vi "View.vi"(0 "object in":refnum<class "Excel.lvclass">, 2 "Requirements":T2, 5 "Error In":errorcluster) -> (14 "object out":refnum<class "Excel.lvclass">, 16 "Message":T1, 19 "Error Out":errorcluster)   [LabVIEW 2024, in "Excel.lvclass"]
doc: "Opens an Excel file and runs Viewer classes Execute method"
uses:
  Excel.lvclass
  Support/Type Def/Requirements.ctl
  Support/Type Def/File Type.ctl
  Support/Type Def/Message.ctl
  IDataMethod_interface/IDataMethod.lvclass
panel:
  # "Connector Pane"
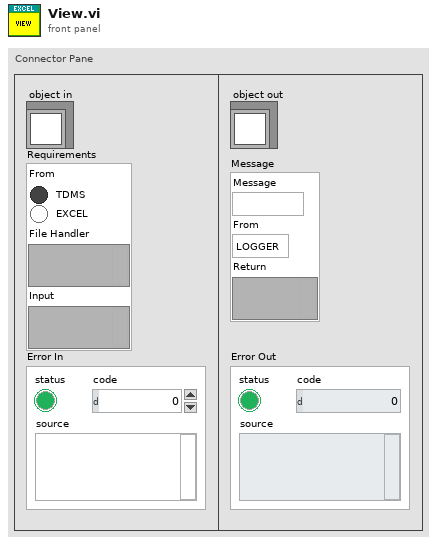
[diagram p1: front panel]
types:
  T1 = typedef "Message.ctl" = cluster{"Message":string, "From":enum16{"LOGGER", "VIEWER"}, "Return":variant}
  T2 = typedef "Requirements.ctl" = cluster{"From":T3, "File Handler":variant, "Input":variant}
  T3 = typedef "File Type.ctl" = enum32{"TDMS", "EXCEL"}
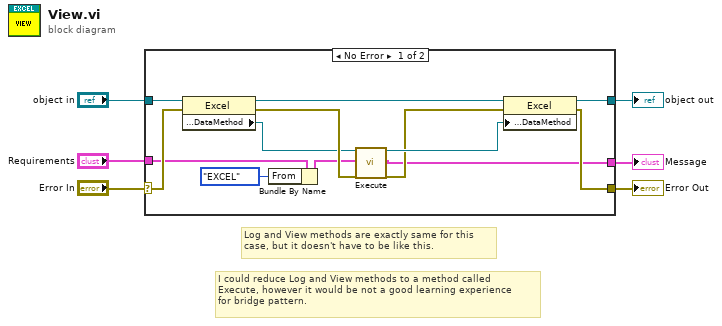
[diagram p0: block diagram]
diagram:
  # "I could reduce Log and View methods to a method called\nExecute, however it would be not a good learning experience\nfor bridge pattern."
  # "Log and View methods are exactly same for this\ncase, but it doesn't have to be like this."
  n1 = case shown="No Error" "Error In" {
    selector: "Error In" -> [w16 w21]
    tunnel: [w15 w21] -> w5
    tunnel: [w17 w20] -> w3
    tunnel: "object in" -> [w19 w20]
    tunnel: "Requirements" -> [w10 _]
    tunnel: [w7 _] -> w1
    frame No Error {
      n2 = property class="Excel"(reference=w19, error in=w16) -> (reference out=w18:refnum<class "Excel.lvclass">, error out=w14:errorcluster, "properties:DataMethod"=w13:refnum<class "IDataMethod.lvclass">)
      n3 = Bundle By Name(cluster=w10, "From"=enum16{"TDMS", "EXCEL"}."EXCEL") -> (w9:T2)
      n4 = call-dynamic "Execute.vi"("object in"=w13, "Requirements"=w9, "Error In"=w14) -> ("object out"=w12:refnum<class "IDataMethod.lvclass">, "Message"=w7:T1, "Error Out"=w11:errorcluster)  [unwired: 14 in]
      n5 = property class="Excel"(reference=w18, error in=w11, "properties:DataMethod"=w12) -> (reference out=w17:refnum<class "Excel.lvclass">, error out=w15:errorcluster)
    }
    frame Error {
    }
  }
  "Error Out" <- w5
  "object out" <- w3
  "Message" <- w1
